vi "Initialise Inside Process.vi"(8 "error in (no error)":errorcluster, 10 "Process":refnum<vi>, 11 "Actor in":refnum<class "Logger Actor.lvclass">) -> (0 "error out":errorcluster, 3 "Actor out":refnum<class "Logger Actor.lvclass">, 5 "Observers":cluster{"Mailbox":refnum<event-registration>})   [LabVIEW 2020, in "Logger Actor.lvclass"]
uses:
  Logger Actor.lvclass
  C:/dev/PGS/2001 - TBCM/Source/RT/RTAF/Source/RTAF/Actors/Base Actor/Actor/Actor.lvclass
  Base Actor/Actor/Message.ctl
  Utility/Log/Log.lvclass
  Logger Actor.lvclass/Logger Actor.ctl
  Base Actor/Actor/Actor.lvclass
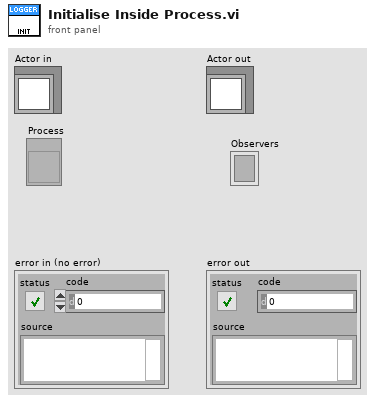
[diagram p1: front panel]
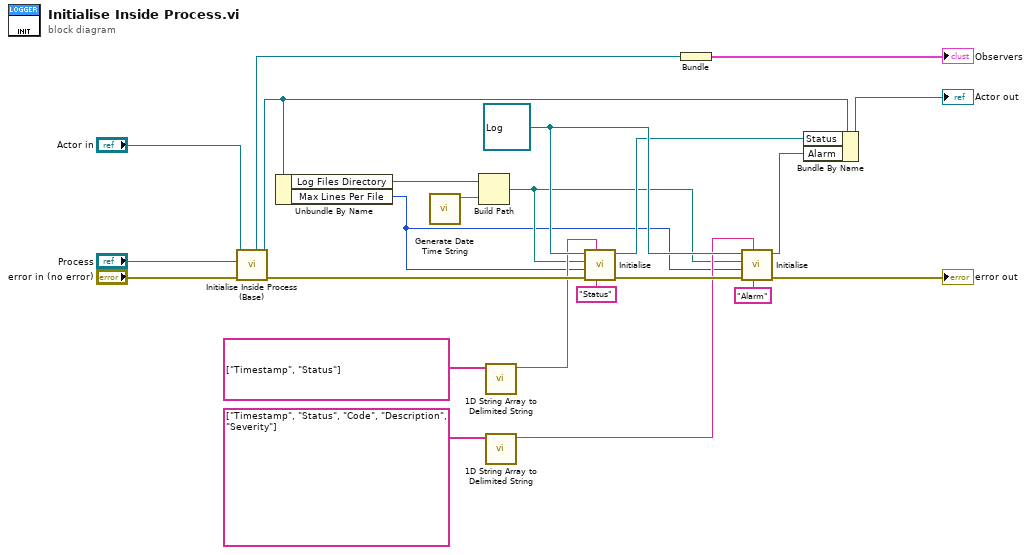
[diagram p0: block diagram]
diagram:
  w21 = refnum<class "Log.lvclass"> refnum ("Log in")
  n1 = call "Initialise Inside Process (Base).vi"("error in (no error)"="error in (no error)", "Process"="Process", "Actor in"="Actor in") -> ("error out"=w15:errorcluster, "Actor out"=w20:refnum<class "Logger Actor.lvclass">, "Mailbox"=w11:refnum<event-registration>)  [unwired: 6 in]
  n2 = Unbundle By Name(w20) -> ("Log Files Directory"=w4:path, "Max Lines Per File"=w2:i32)
  n3 = call "Generate Date Time String.vi"() -> ("Date time string"=w1:string)  [unwired: 10 in, 1 out]
  n4 = Build Path(base path=w4, name or relative path=w1) -> (appended path=w3:path)
  n5 = call <vilib>:"1D String Array to Delimited String.vi"("string array"=string[] ["Timestamp", "Status"]) -> ("delimited string"=w8:string)  [unwired: 10 in]
  n6 = call <vilib>:"1D String Array to Delimited String.vi"("string array"=string[] ["Timestamp", "Status", "Code", "Description", "Severity"]) -> ("delimited string"=w6:string)  [unwired: 10 in]
  n7 = call "Initialise.vi"("Filename"="Status", "Header"=w8, "error in (no error)"=w15, "Max Records"=w2, "Directory"=w3, "Log in"=w21) -> ("error out"=w16:errorcluster, "Log out"=w19:refnum<class "Log.lvclass">)  [unwired: 4 in]
  n8 = Bundle("Mailbox"=w11) -> (→"Observers":cluster{"Mailbox":refnum<event-registration>})  [unwired: 1 in]
  n9 = call "Initialise.vi"("Filename"="Alarm", "Header"=w6, "error in (no error)"=w16, "Max Records"=w2, "Directory"=w3, "Log in"=w21) -> ("error out"=→"error out":errorcluster, "Log out"=w18:refnum<class "Log.lvclass">)  [unwired: 4 in]
  n10 = Bundle By Name(cluster=w20, "Status"=w19, "Alarm"=w18) -> (→"Actor out":refnum<class "Logger Actor.lvclass">)
